vi "BallShear_PackageCapture.vi"(8 "Capture":bool, 9 "Default Image Path":path=path "C:/Users/Nicole/Documents/GitHub/Ball_Shear/0_BallShear/img/default.jpg", 10 "Python Script Path":path=path "C:/Users/Nicole/Documents/GitHub/Ball_Shear/0_BallShear/scripts/livefeed.py", 11 "Target Image Path":path=path "C:/Users/Nicole/Documents/GitHub/Ball_Shear/0_BallShear/img/package.jpg") -> (0 "Success":bool, 3 "Actual Image Path":path)   [LabVIEW 2013]
panel:
  out "standard error":string
  out "concatenated string":string
  out "standard output":string
  out "return code":i32
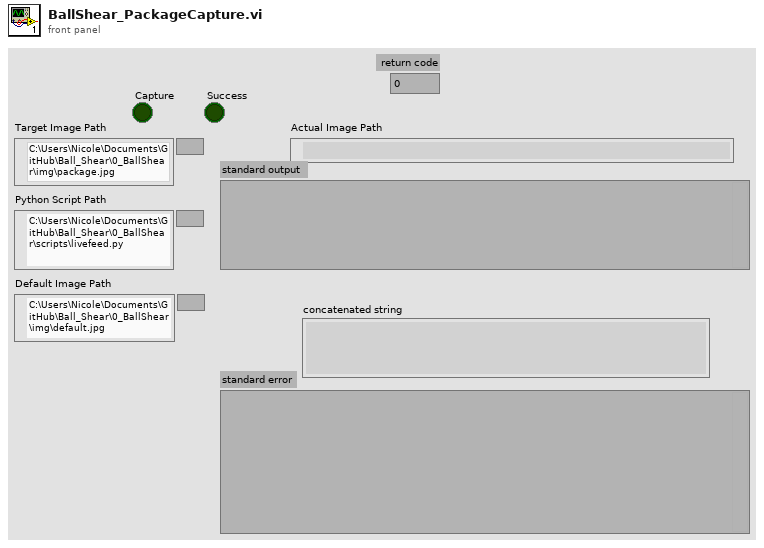
[diagram p1: front panel]
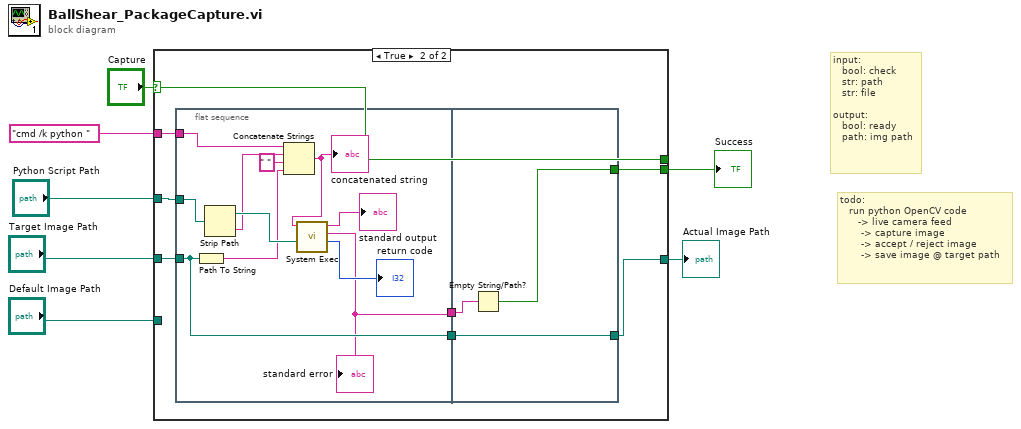
[diagram p0: block diagram]
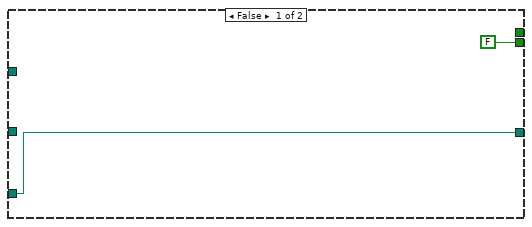
[diagram p2: hidden frame]
diagram:
  # "todo:\n   run python OpenCV code\n      -> live camera feed\n       -> capture image\n       -> accept / reject image\n       -> save image @ target path"
  # "input: \n   bool: check\n   str: path\n   str: file\n\noutput:\n   bool: ready\n   path: img path"
  n1 = case shown="True" "Capture" {
    tunnel: "Capture" -> [_ _]
    tunnel: [FALSE ("Power") w10] -> w6
    tunnel: "Target Image Path" -> [_ w15]
    tunnel: [w8 w12] -> w4
    tunnel: "Python Script Path" -> [_ w16]
    tunnel: "Default Image Path" -> [w8 _]
    tunnel: "cmd /k python " -> [_ w14]
    frame False {
    }
    frame True {
      n2 = flat-sequence {
        tunnel: w16 -> [w27]
        tunnel: w15 -> [w21]
        tunnel: w14 -> [w25]
        tunnel: [w21] -> w13
        tunnel: [w17] -> w11
        tunnel: w13 -> [w30]
        tunnel: [w30] -> w12
        tunnel: w11 -> [w29]
        tunnel: [w28] -> w10
        frame #0 {
          n3 = Path To String(path=w21) -> (string=w19:string)
          n4 = Strip Path(path=w27) -> (stripped path=w26:path, name=w20:string)
          n5 = Concatenate Strings(w25, w20, " " ("string"), w19) -> (w24:string)
          "concatenated string" <- w24
          n6 = call <vilib>:"System Exec.vi"("working directory"=w26, "command line"=w24) -> ("return code"=→"return code":i32, "standard error"=w17:string, "standard output"=→"standard output":string)  [unwired: 6 in, 1 out]
          "standard error" <- w17
        }
        frame #1 {
          n7 = Empty String/Path?(string/path=w29) -> (empty?=w28:bool)
        }
      }
    }
  }
  "Actual Image Path" <- w4
  "Success" <- w6
